vi "Rem_Multi_Array_Elements(DBL).vi"(0 "Input array":dbl[](array[numeric])=[1.0, 2.0, 3.0, 0.0, 0.0, 6.0, 7.0], 3 "Indices to be deleted":i32[](array[numeric])=[1, 2, 3, 0, 0, 6, 7]) -> (6 "Array with elements removed":dbl[](array[numeric]))   [LabVIEW 2011]
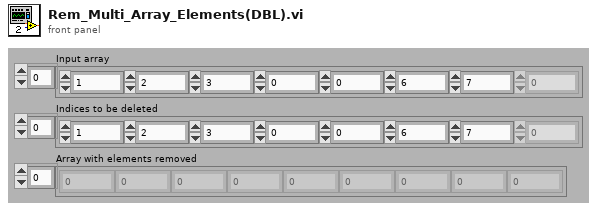
[diagram p1: front panel]
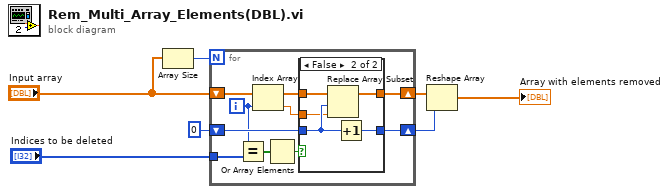
[diagram p0: block diagram]
diagram:
  n1 = Array Size(array="Input array") -> (size(s)=w7:i32)
  n2 = for {
    N: w7 -> [_]
    shift-right: [w16] -> w5
    shift-left: "Input array" -> [w15]
    shift-right: [w13] -> w4
    shift-left: 0 -> [w14]
    tunnel: "Indices to be deleted" -> [w9]
    i -> [w10]
    n3 = Equal?(x=w10, y=w9) -> (x = y?=w11:bool[])
    n4 = Index Array(array=w15, index=w10) -> (element=w12:dbl)
    n5 = Or Array Elements(Boolean array=w11) -> (logical OR=w8:bool)
    n6 = case shown="False" w8 {
      tunnel: w15 -> [w18 w23]
      tunnel: [w18 w22] -> w16
      tunnel: w14 -> [w17 w21]
      tunnel: [w17 w20] -> w13
      tunnel: w12 -> [_ w19]
      frame True {
      }
      frame False {
        n7 = Replace Array Subset(array=w23, new element=w19, index=w21) -> (w22:dbl[])
        n8 = Increment(x=w21) -> (x+1=w20:i32)
      }
    }
  }
  n9 = Reshape Array(w5, w4) -> (→"Array with elements removed":dbl[])
